vi "INTEGRATION TEST - Integrated test.vi"(8 "error in (no error)":errorcluster) -> (0 "error out":errorcluster, 2 "Passed":bool)   [LabVIEW 2020]
uses:
  <vilib>/addons/_JKI Toolkits/Caraya/classes/Assert/Assert True.vi
  <vilib>/Utility/config.llb/NI_LVConfig.lvlib
  <userlib>/_OpenG.lib/file/file.llb/openg_file.lvlib
  <vilib>/addons/_JKI Toolkits/Caraya/classes/Test/Test.lvclass
  <vilib>/addons/_JKI Toolkits/Caraya/classes/Assert/Assert.lvclass
panel:
  out "character string":string
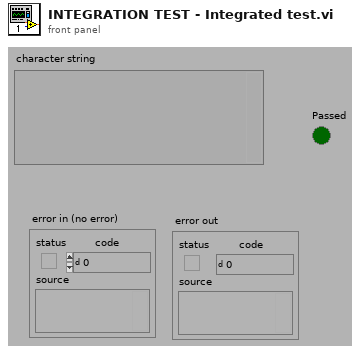
[diagram p1: front panel]
types:
  T1 = typedef "NI_LVConfig.lvlib/Config Data RefNum.ctl" = refnum<k1>
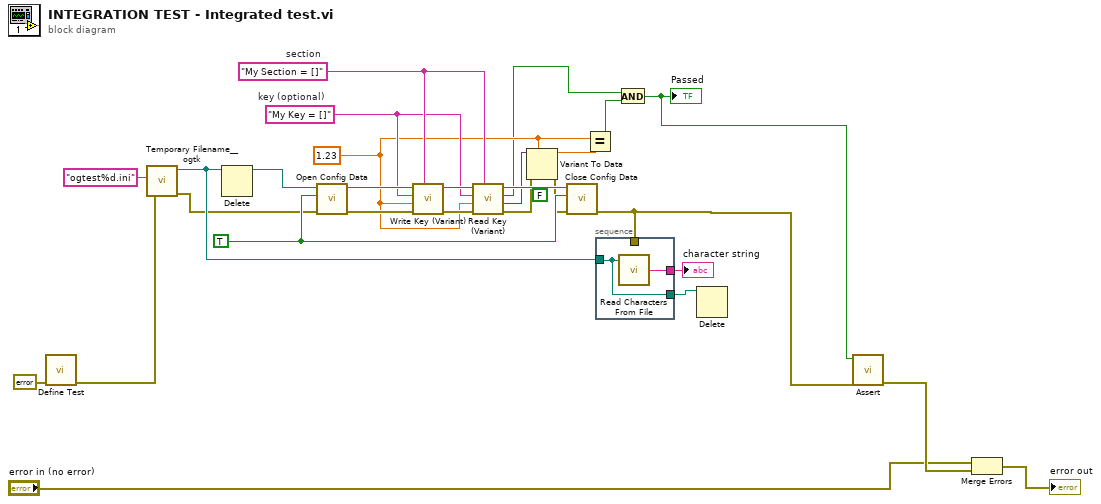
[diagram p0: block diagram]
diagram:
  (unwired) FALSE ("write configuration file? (T)")
  w15 = 1.23 ("Numeric")
  w23 = "My Key = []"  # key (optional)
  w24 = "My Section = []"  # section
  w21 = TRUE ("create file if necessary? (T)")
  n1 = call <vilib>:"Define Test.vi"("error in (no error)"=errorcluster {"status"=FALSE, "code"=0, "source"=""}) -> ("error out"=w5:errorcluster)  [unwired: 9 in, 1 out]
  n2 = call <userlib>:"Temporary Filename__ogtk.vi"("error in (no error)"=w5, "pattern (lvtemp%d.tmp)"="ogtest%d.ini") -> ("error out"=w8:errorcluster, "file in tmp dir"=w9:path)  [unwired: 4 in]
  n3 = Delete(path (use dialog)=w9) -> (deleted path=w16:path)  [unwired: 4 in, 2 out]
  n4 = call <vilib>:"Open Config Data.vi"("error in (no error)"=w8, "create file if necessary (T)"=w21, "configuration file path"=w16) -> ("error out"=w27:errorcluster, "refnum"=w28:T1)  [unwired: 6 in, 1 out]
  n5 = call "Write Key (Variant).vi"("section"=w24, "error in (no error)"=w27, "key-value"=w15, "key (optional)"=w23, "refnum"=w28) -> ("error out"=w25:errorcluster, "refnum out"=w26:T1)  [unwired: 5 in]
  n6 = call "Read Key (Variant).vi"("section"=w24, "error in (no error)"=w25, "type"=w15, "key (optional)"=w23, "refnum"=w26) -> ("error out"=w18:errorcluster, "key-value"=w20:variant, "found?"=w13:bool, "refnum out"=w22:T1)  [unwired: 3 in]
  n7 = Variant To Data(error in=w18, type=w15, Variant=w20) -> (data=w12:dbl, error out=w19:errorcluster)
  n8 = call <vilib>:"Close Config Data.vi"("error in (no error)"=w19, "write file if changed (T)"=w21, "refnum"=w22) -> ("error out"=w4:errorcluster)  [unwired: 7 in, 1 out]
  n9 = Equal?(x=w15, y=w12) -> (x = y?=w14:bool)
  n10 = stacked-sequence {
    tunnel: w9 -> [w29]
    tunnel: [w30] -> w17
    tunnel: w4 -> [_]
    tunnel: [w29] -> w11
    frame #0 {
      n11 = call <vilib>:"Read Characters From File.vi"("file path (dialog if empty)"=w29) -> ("character string"=w30:string)  [unwired: 5 in, 3 out]
    }
  }
  "character string" <- w17
  n12 = And(x=w13, y=w14) -> (x .and. y?=w3:bool)
  "Passed" <- w3
  n13 = Delete(path (use dialog)=w11) -> ()  [unwired: 4 in, 3 out]
  n14 = call-poly <vilib>:"Assert.vi"("error in (no error)"=w4, "True?"=w3) -> ("error out"=w6:errorcluster)  [unwired: 8 in, 1 out]
  n15 = Merge Errors("error in (no error)", w6) -> (→"error out":errorcluster)
